vi "ETPA&TPA.vi"() -> ()   [LabVIEW 2023]
panel:
  in  "number of measurements":i32
  out "number of measurements":i32
  out "Collection Time 2":u32=1000
  out "Function (1: AC Volts)\nFunction(0: DC Volts)":u16=1
  out "counter  2":tag="Dev1/ctr0"
  out "source  2":tag="/Dev1/PFI14"
  out "VISA resource name mulitmeter  2":refnum<visa-resource-name>="sarasMultimeter"
  in  "VISA resource name mulitmeter":refnum<visa-resource-name>
  in  "DEFAULT?":bool
  in  "Collection Time":u32
  in  "Label?":bool
  in  "file path (dialog if empty)":path
  in  "?":bool
  out "PRESENT - COUNTER":dbl(graph)
  out "PRESENT - Multimeter":dbl(graph)
  in  "Function (1: AC Volts)\nFunction(0: DC Volts)":u16
  in  "source":tag
  in  "counter":tag
  out "Current Trial -Multimeter":dbl(graph)
  out "Current Trial - Singles Photon Count Rate":dbl(graph)
  # "Default Settings"
  # "CTR0"
  # "USB0"
  # "PFI14"
  # "Not Default Settings"
  # "PLEASE PUT (\".csv\") at the end of your path"
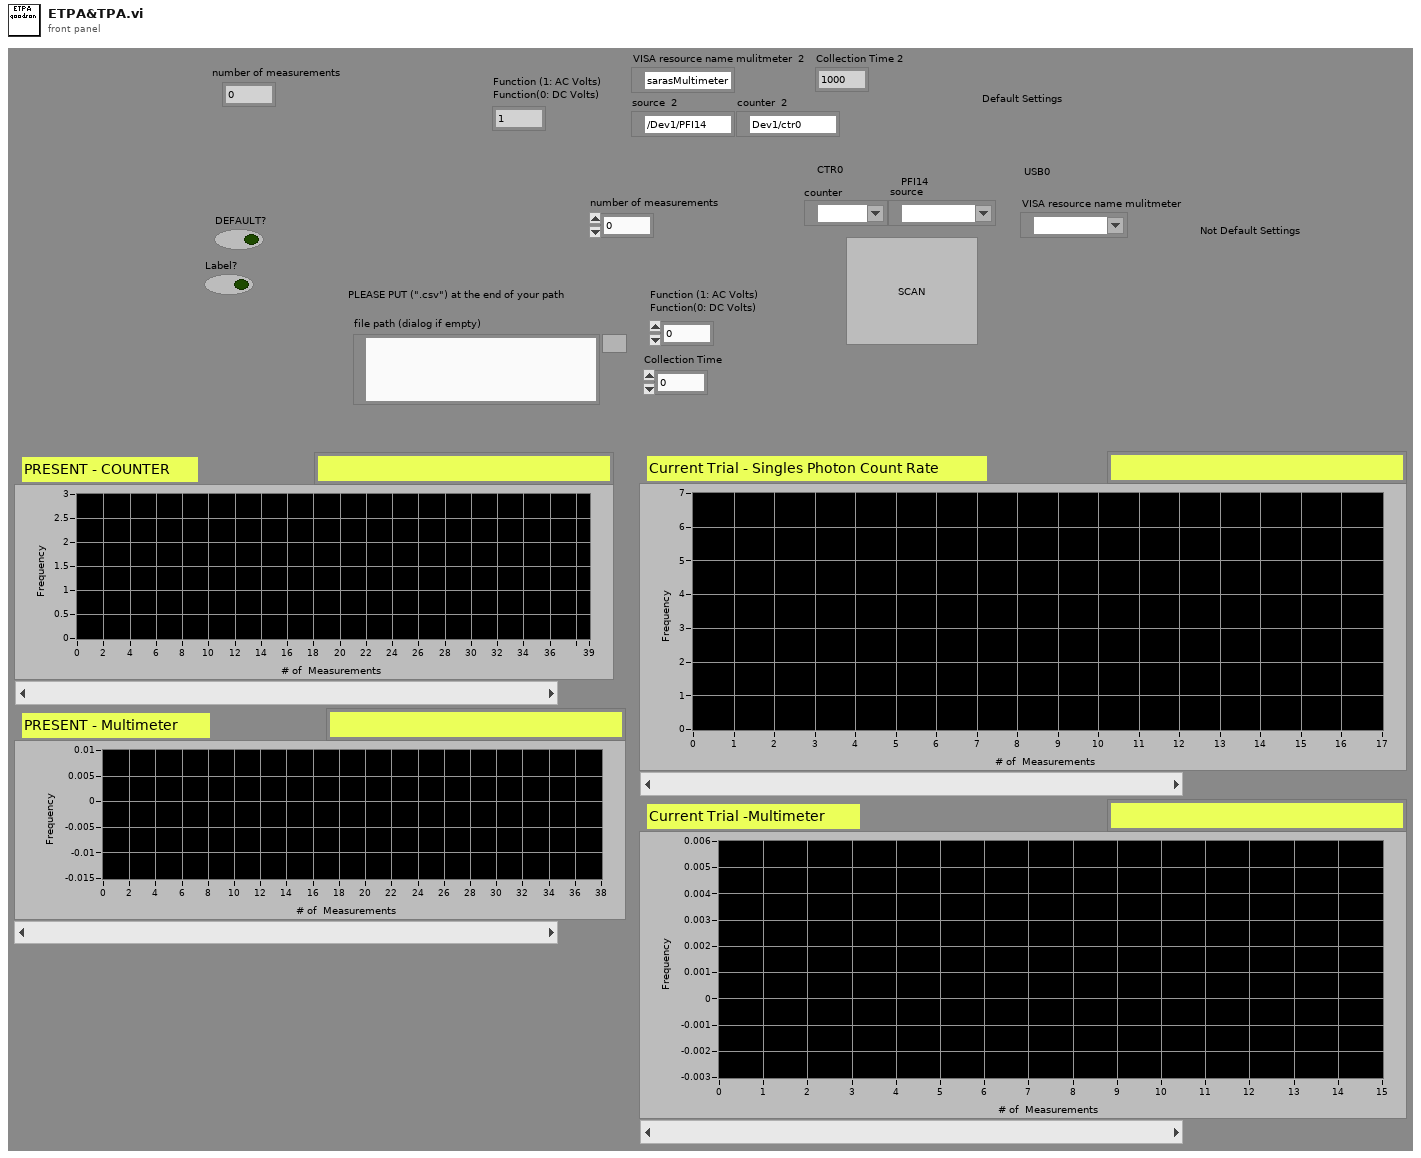
[diagram p1: front panel]
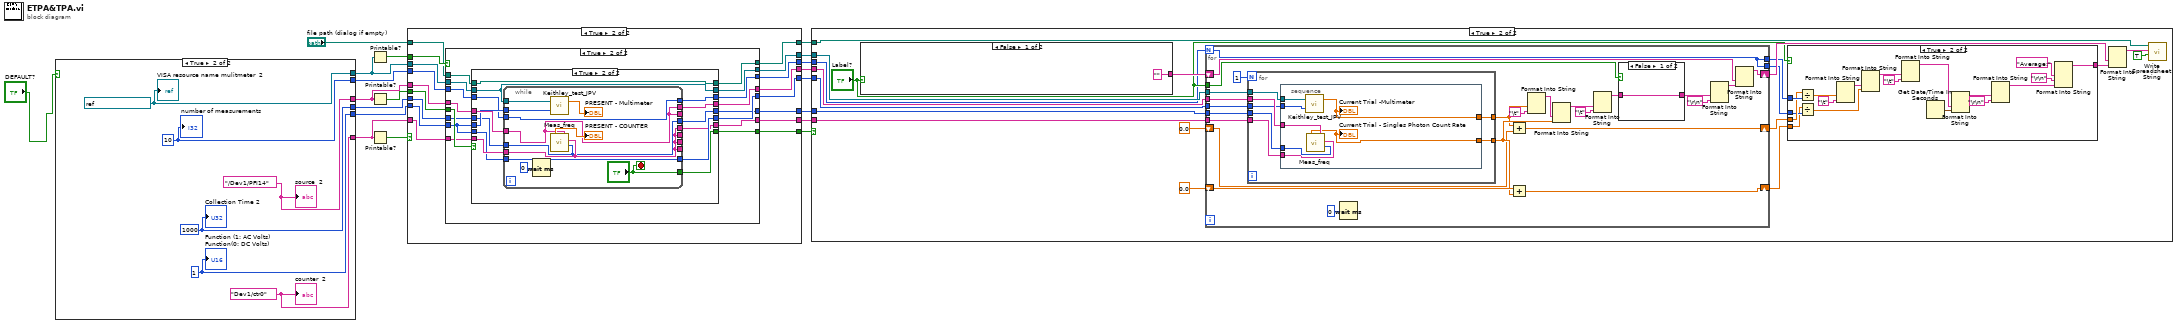
[diagram p0: block diagram]
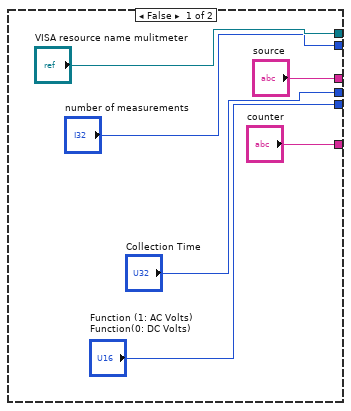
[diagram p2: hidden frame]
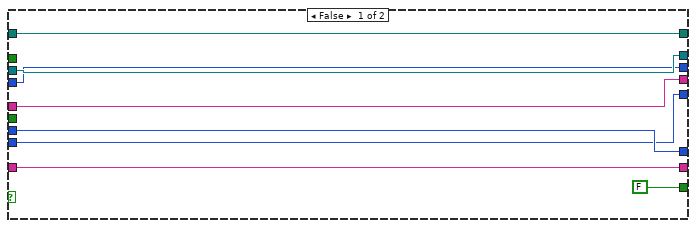
[diagram p3: hidden frame]
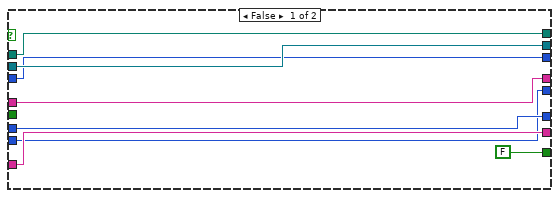
[diagram p4: hidden frame]
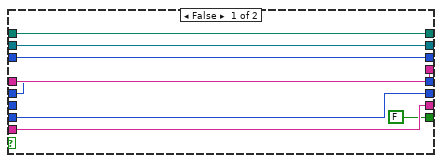
[diagram p5: hidden frame]
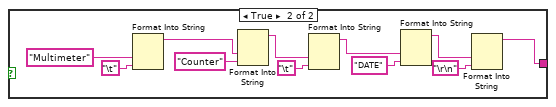
[diagram p7: hidden frame]
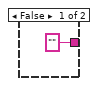
[diagram p8: hidden frame]
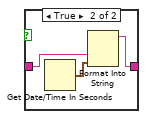
[diagram p9: hidden frame]
diagram:
  n1 = case shown="True" "DEFAULT?" {
    tunnel: ["VISA resource name mulitmeter" w31] -> w7
    tunnel: ["Collection Time" w30] -> w6
    tunnel: ["Function (1: AC Volts)\nFunction(0: DC Volts)" w29] -> w5
    tunnel: ["source" w28] -> w4
    tunnel: ["counter" w27] -> w3
    tunnel: ["number of measurements" w26] -> w1
    frame False {
    }
    frame True {
      w26 = 10
      w27 = tag "Dev1/ctr0" ("counter")
      w28 = tag "/Dev1/PFI14" ("source")
      w29 = u16 1 ("Function (1: AC Volts)\nFunction(0: DC Volts)")
      w30 = u32 1000 ("Collection Time")
      w31 = refnum<visa-resource-name> "sarasMultimeter" ("VISA resource name mulitmeter")
      "VISA resource name mulitmeter  2" <- w31
      "source  2" <- w28
      "counter  2" <- w27
      "Function (1: AC Volts)\nFunction(0: DC Volts)" <- w29
      "Collection Time 2" <- w30
      "number of measurements" <- w26
    }
  }
  n2 = Printable?(1:w7) -> (0:w9:bool)
  n3 = Printable?(1:w4) -> (0:w8:bool)
  n4 = Printable?(1:w3) -> (0:w10:bool)
  n5 = case shown="True" w10 {
    tunnel: w9 -> [_ w56]
    tunnel: w8 -> [_ w55]
    tunnel: w3 -> [w36 w54]
    tunnel: w7 -> [w35 w53]
    tunnel: w4 -> [w37 w52]
    tunnel: w5 -> [w32 w51]
    tunnel: [w37 w50] -> w18
    tunnel: [w35 w49] -> w17
    tunnel: [w32 w48] -> w16
    tunnel: [w36 w47] -> w15
    tunnel: [FALSE w46] -> w14
    tunnel: [w39 w45] -> w13
    tunnel: [w34 w44] -> w12
    tunnel: "file path (dialog if empty)" -> [w39 w43]
    tunnel: w6 -> [w34 w42]
    tunnel: w1 -> [w33 w41]
    tunnel: [w33 w40] -> w2
    frame False {
    }
    frame True {
      n6 = case shown="True" w56 {
        tunnel: w55 -> [_ w80]
        tunnel: w54 -> [w63 w79]
        tunnel: w53 -> [w62 w78]
        tunnel: w52 -> [w64 w77]
        tunnel: w51 -> [w57 w76]
        tunnel: [w64 w75] -> w50
        tunnel: [w62 w74] -> w49
        tunnel: [w57 w73] -> w48
        tunnel: [w63 w72] -> w47
        tunnel: [FALSE w71] -> w46
        tunnel: [w60 w70] -> w45
        tunnel: [w59 w69] -> w44
        tunnel: w43 -> [w60 w68]
        tunnel: w42 -> [w59 w67]
        tunnel: w41 -> [w58 w66]
        tunnel: [w58 w65] -> w40
        frame False {
        }
        frame True {
          n7 = case shown="True" w80 {
            tunnel: [w87 w97] -> w75
            tunnel: [w88 w96] -> w74
            tunnel: [w85 w100] -> w73
            tunnel: [w86 w98] -> w72
            tunnel: [FALSE w95] -> w71
            tunnel: [w83 w92] -> w70
            tunnel: [w82 w99] -> w69
            tunnel: w79 -> [w86 w101]
            tunnel: w78 -> [w88 w96]
            tunnel: w77 -> [w87 w102]
            tunnel: w76 -> [w85 w94]
            tunnel: w76 -> [_ w93]
            tunnel: w68 -> [w83 w92]
            tunnel: w67 -> [w82 w91]
            tunnel: w66 -> [w81 w90]
            tunnel: [w81 w89] -> w65
            frame False {
            }
            frame True {
              n8 = while {
                tunnel: [w109] -> w100
                tunnel: [w107] -> _
                tunnel: [w106] -> w99
                tunnel: [w107] -> _
                tunnel: [w107] -> _
                tunnel: [w105] -> _
                tunnel: w96 -> [w111]
                tunnel: w102 -> [w105]
                tunnel: w101 -> [w107]
                tunnel: [w107] -> w98
                tunnel: [w105] -> w97
                tunnel: ["?"] -> w95
                tunnel: w94 -> [w109]
                tunnel: w93 -> [w108]
                tunnel: w91 -> [w106]
                tunnel: w90 -> [w104]
                tunnel: [w104] -> w89
                stop <- "?" stop-if-true
                n9 = Wait (ms)(milliseconds to wait=u32 0) -> ()  [unwired: 1 out]
                n10 = call "Keithley_test_JPV.vi"("Function (0: DC Volts)"=w108, "VISA resource name"=w111) -> ("Measurement"=→"PRESENT - Multimeter":dbl)  [unwired: 1 out]
                n11 = call "Meas_freq.vi"("source"=w105, "counter"=w107, "Time miliseconds"=w106) -> (0:→"PRESENT - COUNTER":dbl)  [unwired: 1 in]
              }
            }
          }
        }
      }
    }
  }
  n12 = case shown="True" w14 {
    tunnel: w12 -> [_ w132]
    tunnel: w18 -> [_ w131]
    tunnel: w17 -> [_ w130]
    tunnel: w16 -> [_ w129]
    tunnel: w15 -> [_ w128]
    tunnel: w13 -> [_ w127]
    tunnel: w2 -> [_ w114]
    frame False {
    }
    frame True {
      n13 = case shown="False" "Label?" {
        tunnel: ["" w139] -> w126
        frame False {
        }
        frame True {
          n14 = Format Into String("Multimeter" ("input 2"), "\t") -> (resulting string=w143:string)  [unwired: 3 in, 1 out]
          n15 = Format Into String(w143, "Counter" ("input 2")) -> (resulting string=w138:string)  [unwired: 3 in, 1 out]
          n16 = Format Into String(w138, "\t") -> (resulting string=w136:string)  [unwired: 3 in, 1 out]
          n17 = Format Into String(w136, "DATE" ("input 2")) -> (resulting string=w135:string)  [unwired: 3 in, 1 out]
          n18 = Format Into String(w135, "\r\n") -> (resulting string=w139:string)  [unwired: 3 in, 1 out]
        }
      }
      n19 = for {
        N: w114 -> [w181]
        tunnel: w132 -> [w188]
        tunnel: w131 -> [w187]
        tunnel: w130 -> [w186]
        tunnel: w129 -> [w185]
        tunnel: w128 -> [w184]
        shift-right: [w182] -> w125
        shift-left: w126 -> [w183]
        shift-right: [w167] -> w116
        shift-left: 0.0 -> [w172]
        shift-right: [w168] -> w118
        shift-left: 0.0 -> [w169]
        tunnel: [w181] -> w117
        tunnel: [w181] -> w119
        tunnel: "Label?" -> [w166]
        n20 = for {
          N: 1 -> [_]
          tunnel: w188 -> [w199]
          tunnel: w187 -> [w198]
          tunnel: w186 -> [w197]
          tunnel: w185 -> [w196]
          tunnel: w184 -> [w195]
          tunnel: [w194] -> w170
          tunnel: [w193] -> w171
          n21 = stacked-sequence {
            tunnel: w199 -> [w206]
            tunnel: w198 -> [w205]
            tunnel: w197 -> [w204]
            tunnel: w196 -> [w203]
            tunnel: w195 -> [w200]
            tunnel: [w202] -> w194
            tunnel: [w201] -> w193
            frame #0 {
              n22 = call "Keithley_test_JPV.vi"("Function (0: DC Volts)"=w203, "VISA resource name"=w204) -> ("Measurement"=w202:dbl)  [unwired: 1 out]
              "Current Trial -Multimeter" <- w202
              n23 = call "Meas_freq.vi"("source"=w205, "counter"=w200, "Time miliseconds"=w206) -> (0:w201:dbl)  [unwired: 1 in]
              "Current Trial - Singles Photon Count Rate" <- w201
            }
          }
        }
        n24 = Wait (ms)(milliseconds to wait=u32 0) -> ()  [unwired: 1 out]
        n25 = Add(x=w170, y=w169) -> (x+y=w168:dbl)
        n26 = Add(x=w172, y=w171) -> (x+y=w167:dbl)
        n27 = Format Into String(w170, "\t") -> (resulting string=w176:string)  [unwired: 3 in, 1 out]
        n28 = Format Into String(w176, w171) -> (resulting string=w178:string)  [unwired: 3 in, 1 out]
        n29 = Format Into String(w178, "\t") -> (resulting string=w179:string)  [unwired: 3 in, 1 out]
        n30 = case shown="False" w166 {
          tunnel: [w189 w192] -> w180
          tunnel: w179 -> [w189 w191]
          frame False {
          }
          frame True {
            n31 = Get Date/Time In Seconds() -> (seconds since 1Jan1904=w190:timestamp)
            n32 = Format Into String(w191, w190) -> (resulting string=w192:string)  [unwired: 3 in, 1 out]
          }
        }
        n33 = Format Into String(w180, "\r\n") -> (resulting string=w177:string)  [unwired: 3 in, 1 out]
        n34 = Format Into String(w183, w177) -> (resulting string=w182:string)  [unwired: 3 in, 1 out]
      }
      n35 = case shown="True" "Label?" {
        tunnel: ["" w157] -> w120
        tunnel: w119 -> [_ w151]
        tunnel: w118 -> [_ w150]
        tunnel: w117 -> [_ w148]
        tunnel: w116 -> [_ w147]
        frame False {
        }
        frame True {
          n36 = Divide(x=w150, y=w151) -> (x/y=w149:dbl)
          n37 = Divide(x=w147, y=w148) -> (x/y=w146:dbl)
          n38 = Format Into String(w149, "\t") -> (resulting string=w156:string)  [unwired: 3 in, 1 out]
          n39 = Format Into String(w156, w146) -> (resulting string=w155:string)  [unwired: 3 in, 1 out]
          n40 = Format Into String(w155, "\t") -> (resulting string=w152:string)  [unwired: 3 in, 1 out]
          n41 = Get Date/Time In Seconds() -> (seconds since 1Jan1904=w161:timestamp)
          n42 = Format Into String(w152, w161) -> (resulting string=w163:string)  [unwired: 3 in, 1 out]
          n43 = Format Into String(w163, "\r\n") -> (resulting string=w158:string)  [unwired: 3 in, 1 out]
          n44 = Format Into String("Average:" ("input 4"), "\r\n", w158) -> (resulting string=w157:string)  [unwired: 3 in, 1 out]
        }
      }
      n45 = Format Into String(w125, w120) -> (resulting string=w121:string)  [unwired: 3 in, 1 out]
      n46 = call <vilib>:"Write Spreadsheet String.vi"("append to file? (new file:F)"=TRUE, "spreadsheet string"=w121, "file path (dialog if empty)"=w127) -> ()  [unwired: 7 in, 2 out]
    }
  }
